vi "PLC_CODMn 获取仪器状态.vi"() -> (3 "PLC版_CODMn状态":u16(ring) items=["待机", "润洗", "进样", "加草酸钠", "反滴定", "排液"])   [LabVIEW 2016, in "质控单元V2.lvlib"]
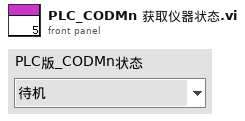
[diagram p1: front panel]
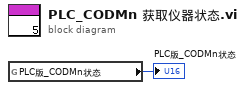
[diagram p0: block diagram]
diagram:
  n1 = global read "系统交互.vi" "PLC版_CODMn状态"() -> (→"PLC版_CODMn状态":u16)
